vi "3_Cross_Correlation_Part_II.vi"(8 "error in (no error)":errorcluster) -> (0 "error out":errorcluster)   [LabVIEW 2014]
uses:
  SwabianInstruments.TimeTagger
panel:
  out "Cross correlation showing <60 ps jitter":cluster{"getIndex":i64[], "getData":i32[]}(graph)
  # "cross correlation between channels 1 and 2\nbinwidth=10 ps, n_bins=400, thus we sample 4 ns\nThe standard deviation of the peak\nis the root mean square sum of the\ninput jitters of channels 1 and 2 we should see the \ncorrelation delta peaks at a bit more than 1000 ns distance"
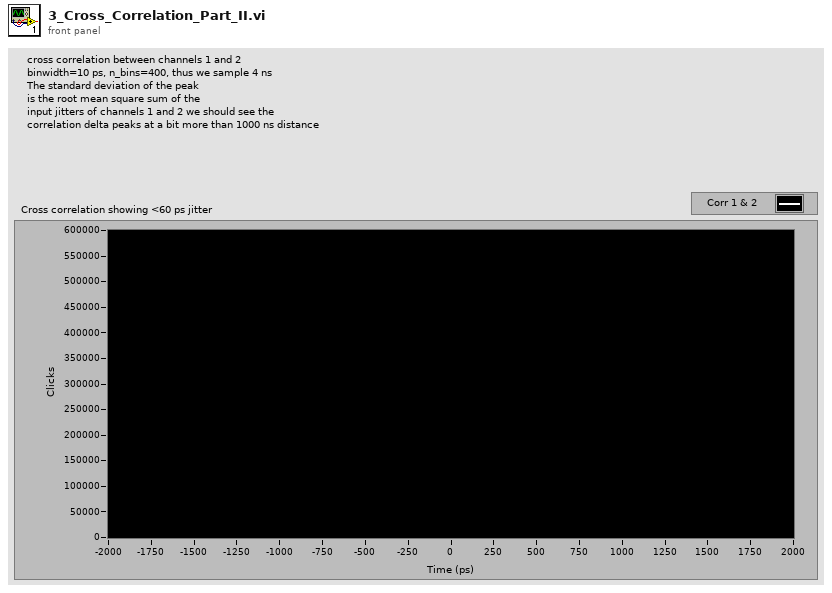
[diagram p1: front panel]
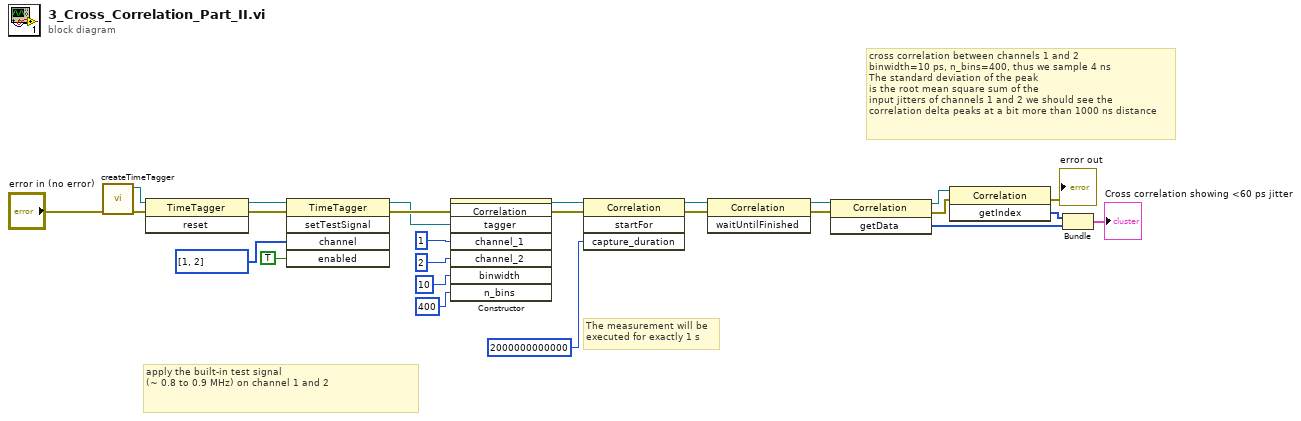
[diagram p0: block diagram]
diagram:
  # "The measurement will be\nexecuted for exactly 1 s"
  # "cross correlation between channels 1 and 2\nbinwidth=10 ps, n_bins=400, thus we sample 4 ns\nThe standard deviation of the peak\nis the root mean square sum of the\ninput jitters of channels 1 and 2 we should see the \ncorrelation delta peaks at a bit more than 1000 ns distance"
  # "apply the built-in test signal\n(~ 0.8 to 0.9 MHz) on channel 1 and 2"
  n1 = call "createTimeTagger.vi"("error in (no error)"="error in (no error)") -> ("error out"=w11:errorcluster, "TimeTagger ref out"=w12:refnum<k24>)  [unwired: 9 in]
  n2 = invoke class="TimeTagger" method="reset"(reference=w12, error in=w11) -> (reference out=w18:refnum<k24>, error out=w19:errorcluster)  [unwired: 1 in, 1 out]
  n3 = invoke class="TimeTagger" method="setTestSignal"(reference=w18, error in=w19, "channel"=i32[] [1, 2], "enabled"=TRUE) -> (reference out=w10:refnum<k24>, error out=w14:errorcluster)  [unwired: 1 in, 3 out]
  n4 = constructor class="Correlation"(error in=w14, "tagger"=w10, "channel_1"=1, "channel_2"=2, "binwidth"=i64 10, "n_bins"=400) -> (reference out=w9:refnum<k24>, error out=w8:errorcluster)  [unwired: 2 in, 6 out]
  n5 = invoke class="Correlation" method="startFor"(reference=w9, error in=w8, "capture_duration"=i64 2000000000000) -> (reference out=w6:refnum<k24>, error out=w4:errorcluster)  [unwired: 1 in, 2 out]
  n6 = invoke class="Correlation" method="waitUntilFinished"(reference=w6, error in=w4) -> (reference out=w5:refnum<k24>, error out=w3:errorcluster)  [unwired: 1 in, 1 out]
  n7 = invoke class="Correlation" method="getData"(reference=w5, error in=w3) -> (reference out=w25:refnum<k24>, error out=w24:errorcluster, "getData"=w15:i32[])  [unwired: 1 in]
  n8 = invoke class="Correlation" method="getIndex"(reference=w25, error in=w24) -> (error out=→"error out":errorcluster, "getIndex"=w16:i64[])  [unwired: 1 in, 1 out]
  n9 = Bundle("getIndex"=w16, "getData"=w15) -> (→"Cross correlation showing <60 ps jitter":cluster{"getIndex":i64[], "getData":i32[]})  [unwired: 1 in]
